vi "Within Percentage.vi"(1 "Allowable Percentage":dbl, 2 "Actual Value":dbl format="%#_13g", 3 "Setpoint":dbl format="%#_13g") -> (0 "Within Allowable %":bool)   [LabVIEW 2018]
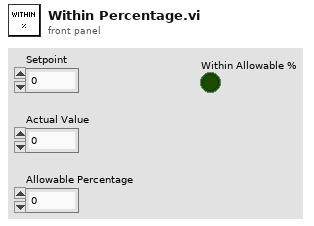
[diagram p1: front panel]
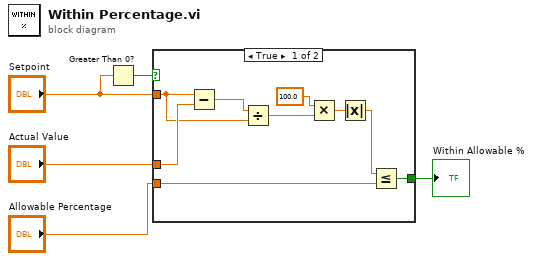
[diagram p0: block diagram]
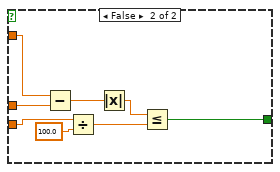
[diagram p2: hidden frame]
diagram:
  n1 = Greater Than 0?(x="Setpoint") -> (x > 0?=w3:bool)
  n2 = case shown="True" w3 {
    tunnel: "Allowable Percentage" -> [w9 w17]
    tunnel: "Actual Value" -> [w8 w20]
    tunnel: "Setpoint" -> [w7 w19]
    tunnel: [w6 w18] -> w1
    frame True {
      n3 = Subtract(x=w7, y=w8) -> (x-y=w14:dbl)
      n4 = Divide(x=w14, y=w7) -> (x/y=w12:dbl)
      n5 = Multiply(x=100.0, y=w12) -> (x*y=w10:dbl)
      n6 = Absolute Value(x=w10) -> (abs(x)=w13:dbl)
      n7 = Less Or Equal?(x=w13, y=w9) -> (x <= y?=w6:bool)
    }
    frame False {
      n8 = Subtract(x=w19, y=w20) -> (x-y=w21:dbl)
      n9 = Divide(x=w17, y=100.0) -> (x/y=w15:dbl)
      n10 = Absolute Value(x=w21) -> (abs(x)=w22:dbl)
      n11 = Less Or Equal?(x=w22, y=w15) -> (x <= y?=w18:bool)
    }
  }
  "Within Allowable %" <- w1
